vi "configure stimulation dialog (subVI).vi"(7 "default directory (none)":path, 8 "error in (no error)":errorcluster, 9 "use initial config? (F)":bool, 10 "odor and manifold config":T1, 11 "initial stim. config [] (empty array)":T11 {"right odor"."port-odor ring" items=["off"=0, "fish water, 3 <Odor:3, Port:0>"=3, "alarm substance <Odor:5, Port:1>"=5]; "middle odor"."port-odor ring" items=["off"=0, "fish water, 2 <Odor:2, Port:0>"=2]; "left odor"."port-odor ring" items=["off"=0, "fish water, 1 <Odor:1, Port:0>"=1, "alanine <Odor:4, Port:1>"=4]; "duration, s" format="%.1f"}) -> (0 "error out":errorcluster, 2 "operation failed?":bool, 3 "stim. config [] out":T11 {"right odor"."port-odor ring" items=["off"=0, "fish water, 3 <Odor:3, Port:0>"=3, "alarm substance <Odor:5, Port:1>"=5]; "middle odor"."port-odor ring" items=["off"=0, "fish water, 2 <Odor:2, Port:0>"=2]; "left odor"."port-odor ring" items=["off"=0, "fish water, 1 <Odor:1, Port:0>"=1, "alanine <Odor:4, Port:1>"=4]; "duration, s" format="%.1f"})   [LabVIEW 2021]
uses:
  type-defs/stimulation configuration array (type def).ctl
  type-defs/stimulator configuration line cluster (type def).ctl
  type-defs/port-odor with color cluster (type def).ctl
  type-defs/port-odor ring (type def).ctl
  type-defs/odor color (type def).ctl
  type-defs/odor and manifold config cluster (type def).ctl
  type-defs/manifold configuration cluster array (type def).ctl
  type-defs/manifold configuration cluster (type def).ctl
  type-defs/manifold selection.ctl
  type-defs/single port single odor cluster.ctl
  type-defs/port number (type def).ctl
  type-defs/odor selection (type def).ctl
  type-defs/odor description array (type def).ctl
  type-defs/odor info cluster (type def).ctl
  type-defs/stimulation config UI states (type def).ctl
  type-defs/project_custom_error_codes_ring (type def).ctl
  <vilib>/Utility/error.llb/DialogType.ctl
  global-variables/global variables.vi
  <vilib>/Utility/error.llb/Error Cluster From Error Code.vi
  <vilib>/ErrorRing/Error Ring.xnode
panel:
  in  "stim. config array dialog":T11 caption="Configure Odor Stimulation Sequence" {"right odor"."port-odor ring" items=["off"=0, "fish water, 3 (Odor: 3, Port: R.1)"=3, "alarm substance (Odor: 5, Port: R.2)"=5]; "middle odor"."port-odor ring" items=["off"=0, "fish water, 2 (Odor: 2, Port: M.1)"=2]; "left odor"."port-odor ring" items=["off"=0, "fish water, 1 (Odor: 1, Port: L.1)"=1, "alanine (Odor: 4, Port: L.2)"=4]; "duration, s" format="%.1f"}
  out "value error source":string
  in  "load config":bool
  in  "save config":bool
  in  "confirm button":bool
  in  "cancel button":bool
  # "description"
  # "duration, s"
  # "left"
  # "middle"
  # "right"
  # "File"
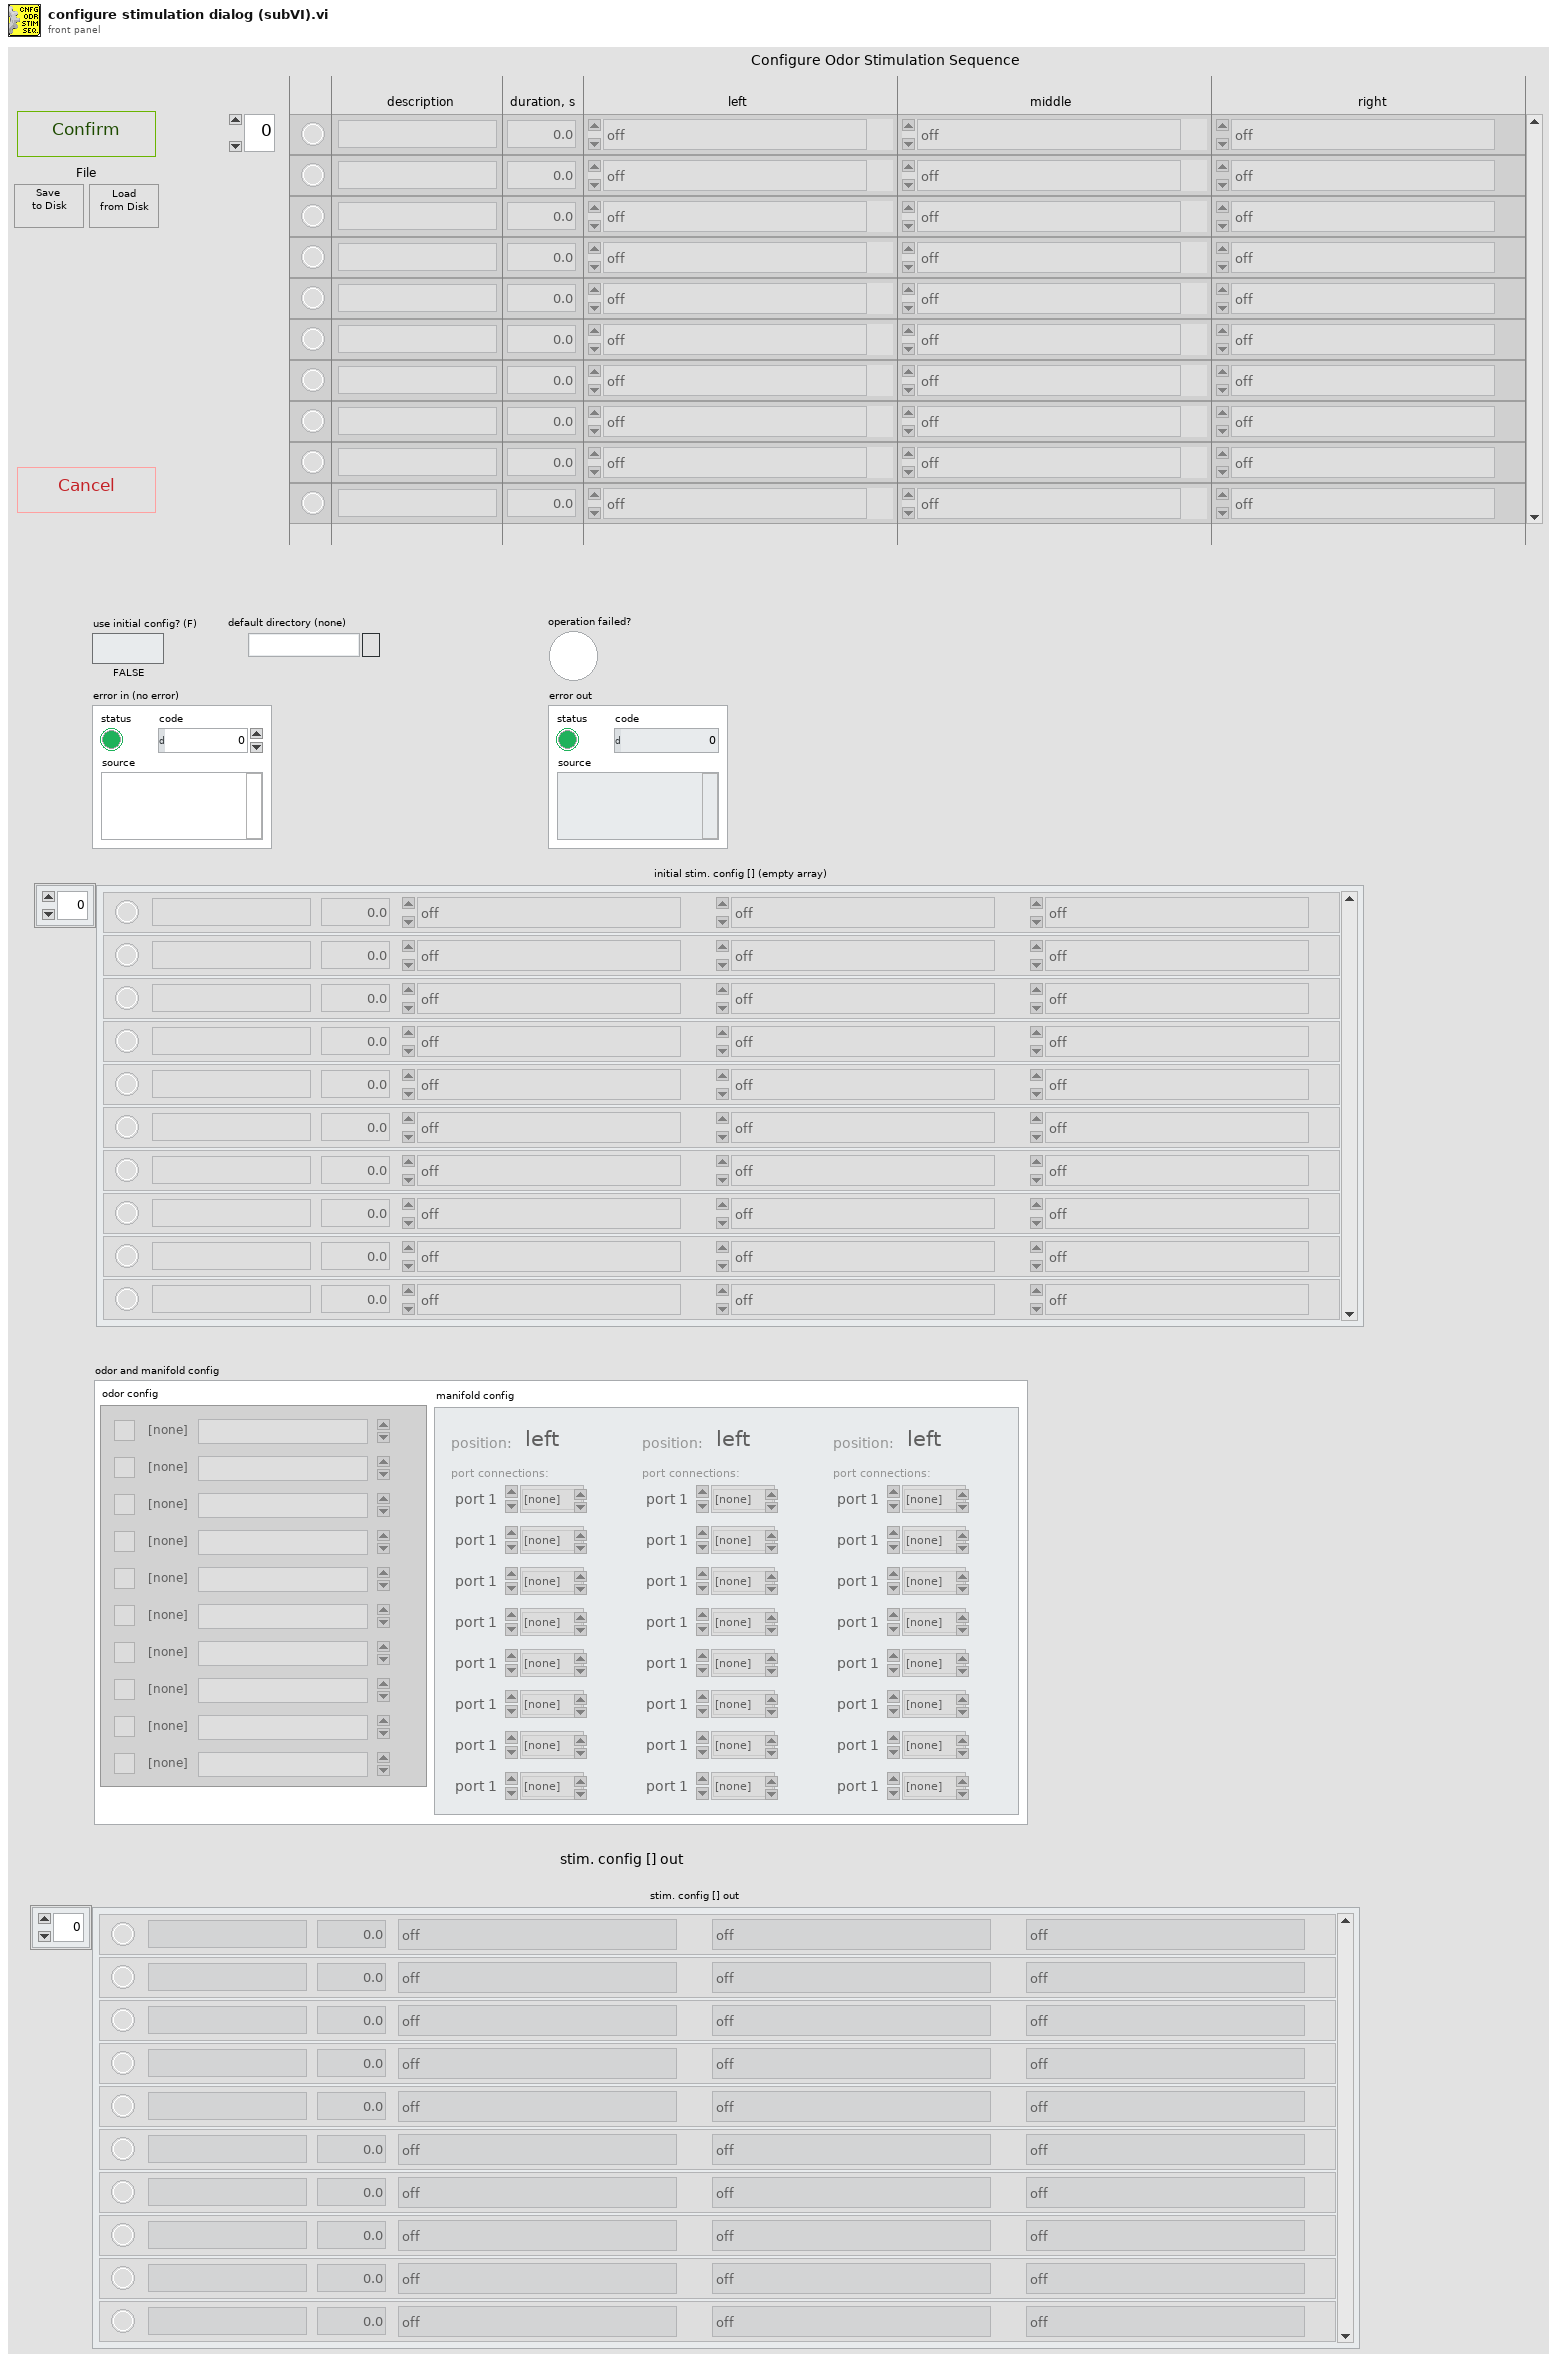
[diagram p1: front panel]
types:
  T1 = typedef "odor and manifold config cluster (type def).ctl" = cluster{"manifold config":T2, "odor config":T9}
  T2 = typedef "manifold configuration cluster array (type def).ctl" = T3[]
  T3 = typedef "manifold configuration cluster (type def).ctl" = cluster{"position:":T4, "port connections:":T5[]}
  T4 = typedef "manifold selection.ctl" = enum16{"left", "middle", "right"}
  T5 = typedef "single port single odor cluster.ctl" = cluster{"port number":T6, "connected odor":T7, "error":bool, "odor color":T8}
  T6 = typedef "port number (type def).ctl" = enum16{"port 1", "port 2", "port 3", "port 4", "port 5", "port 6", "port 7", "port 8"}
  T7 = typedef "odor selection (type def).ctl" = enum16{"[none]", "odor 1", "odor 2", "odor 3", "odor 4", "odor 5", "odor 6", "odor 7", "odor 8", "odor 9", "odor 10"}
  T8 = typedef "odor color (type def).ctl" = u16
  T9 = typedef "odor description array (type def).ctl" = T10[]
  T10 = typedef "odor info cluster (type def).ctl" = cluster{"odor channel":T7, "odor description":string, "odor color":T8, "odor channel active":bool}
  T11 = typedef "stimulation configuration array (type def).ctl" = T12[]
  T12 = typedef "stimulator configuration line cluster (type def).ctl" = cluster{"description":string, "duration, s":dbl, "left odor":T13, "middle odor":T13, "right odor":T13, "selected?":bool}
  T13 = typedef "port-odor with color cluster (type def).ctl" = cluster{"port-odor ring":T14, "odor color":T8}
  T14 = typedef "port-odor ring (type def).ctl" = u16
  T15 = typedef "stimulation config UI states (type def).ctl" = enum16{"Initialize", "Wait For Event", "Open Odor-Manifold Dialog", "Update Stim Config", "Handle Errors", "Save Config to File", "Load Config from File", "Exit", "Crash"}
  T16 = enum8{"Enabled", "Disabled", "Disabled and Grayed Out"}
  T17 = enum16{"open", "replace", "create", "open or create", "replace or create", "replace or create with confirmation"}
  T18 = enum16{"big-endian, network order", "native, host order", "little-endian"}
  T19 = cluster{"stim. config line cluster":refnum<vi>, "description string":refnum<vi>, "duration, s numeric":refnum<vi>, "port-odor & color cluster []":refnum<vi>[], "port-odor ring []":refnum<vi>[], "odor color ring []":refnum<vi>[]}
  T20 = typedef "project_custom_error_codes_ring (type def).ctl" = i32
  T21 = typedef "DialogType.ctl" = u16
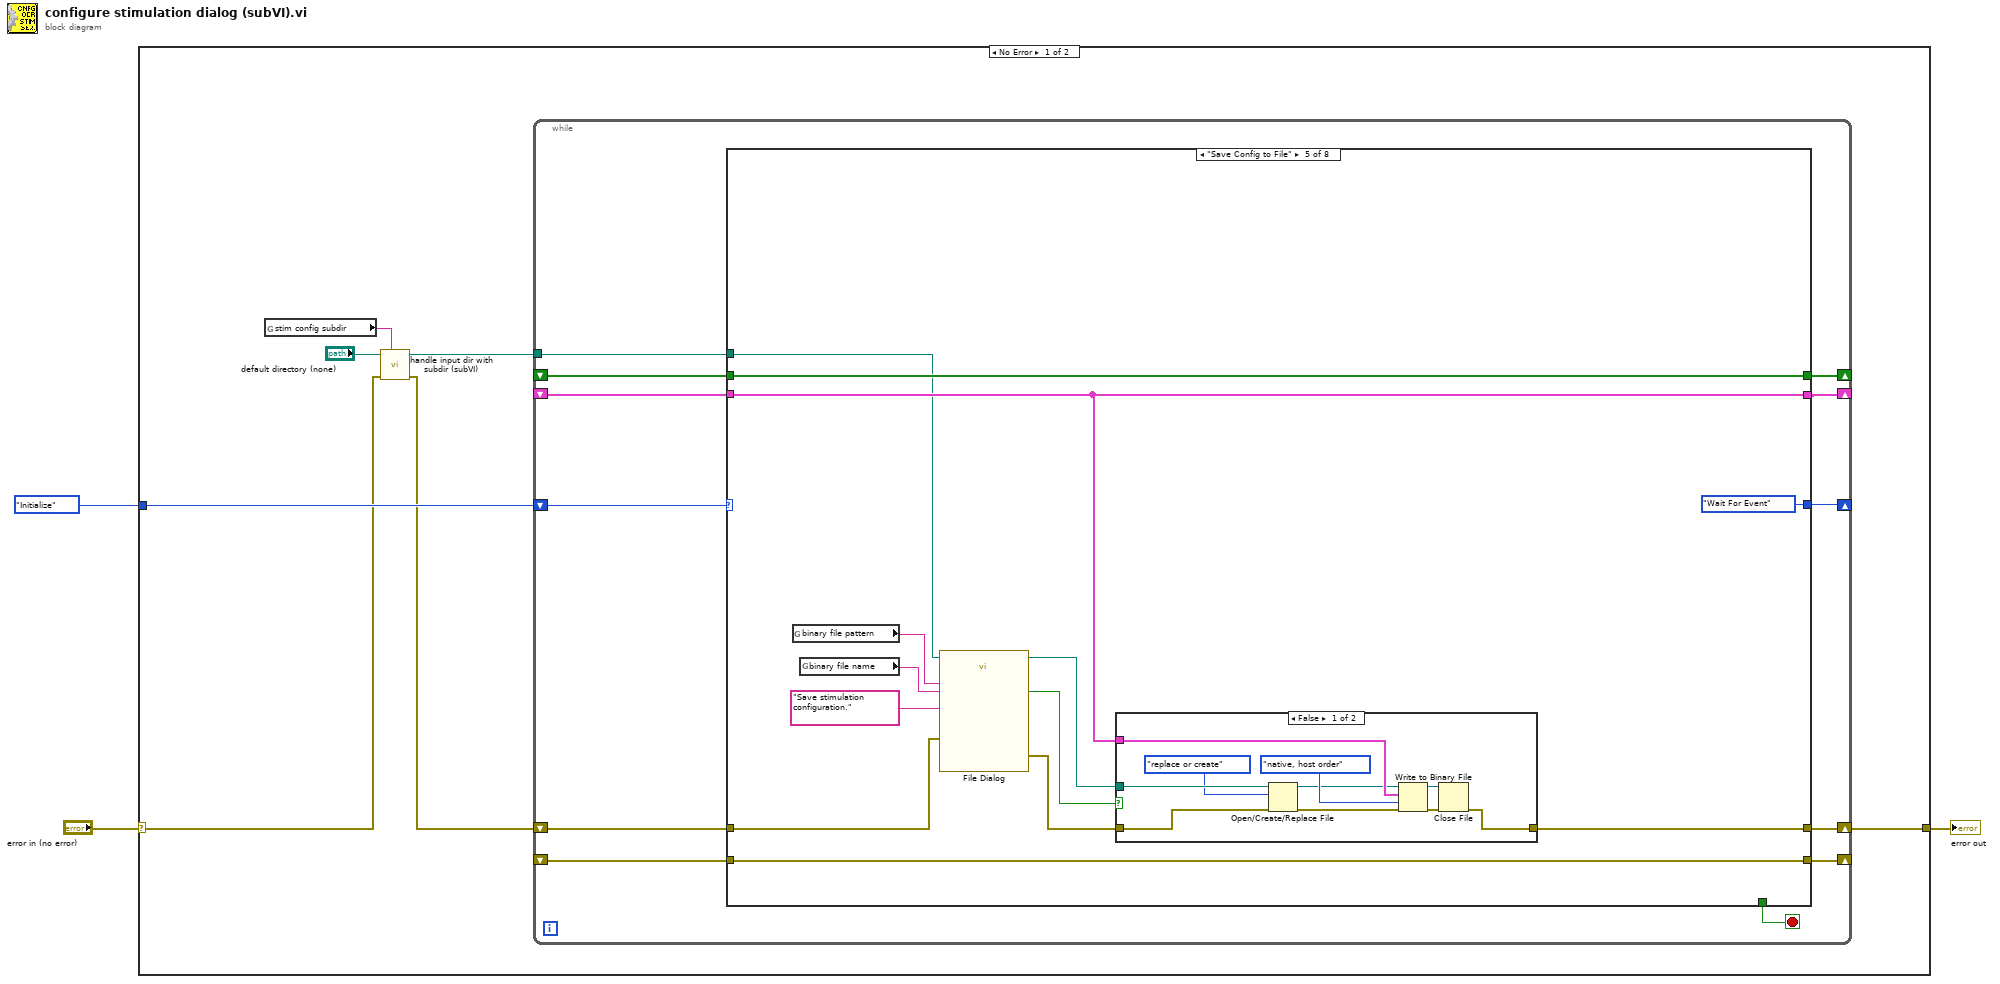
[diagram p0: block diagram]
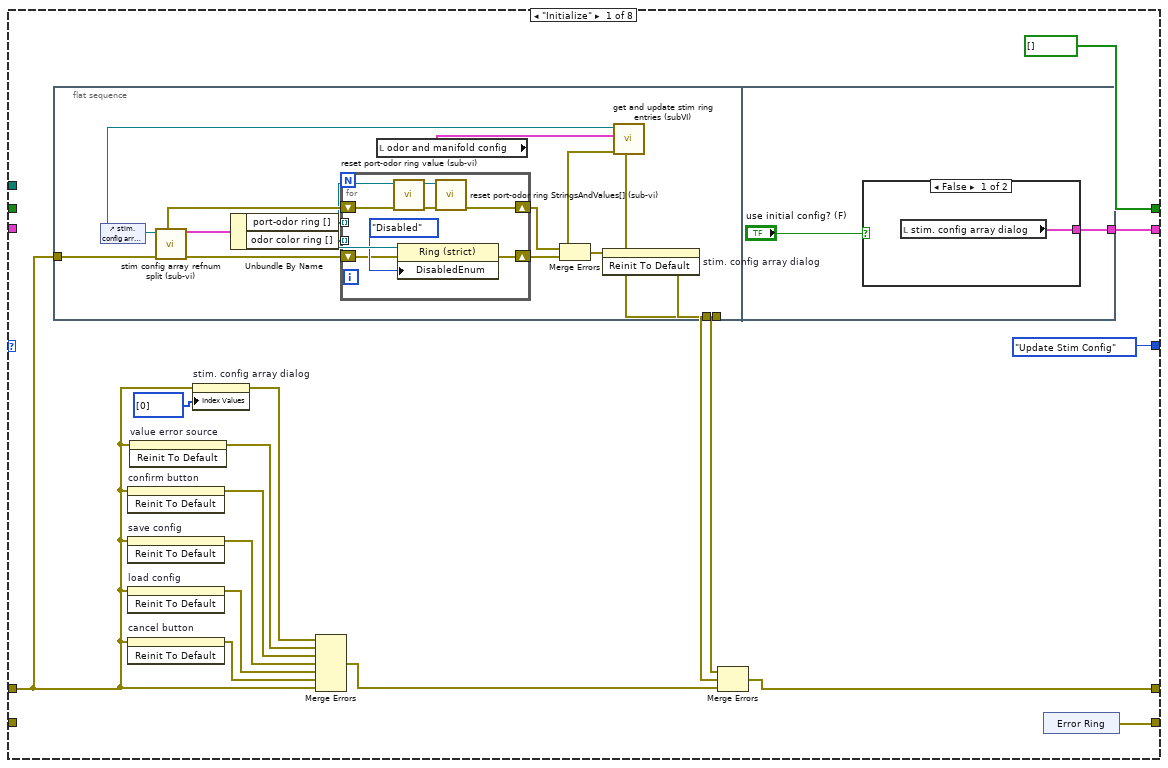
[diagram p2: hidden frame]
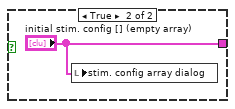
[diagram p3: hidden frame]
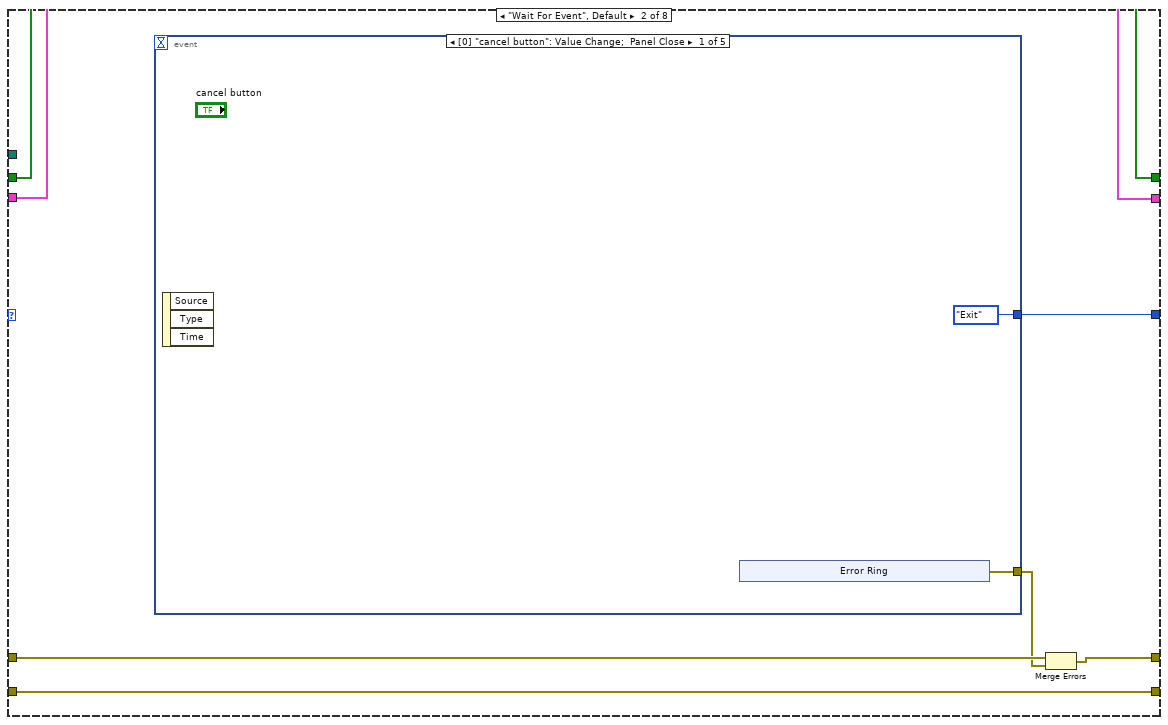
[diagram p4: hidden frame]
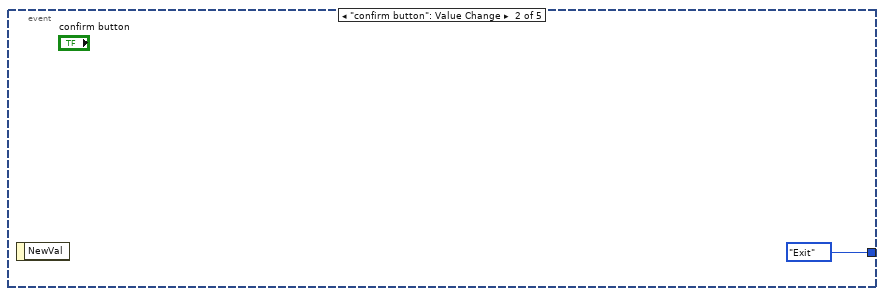
[diagram p5: hidden frame]
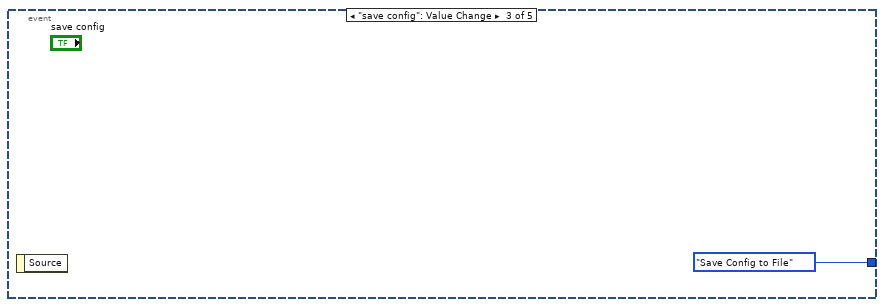
[diagram p6: hidden frame]
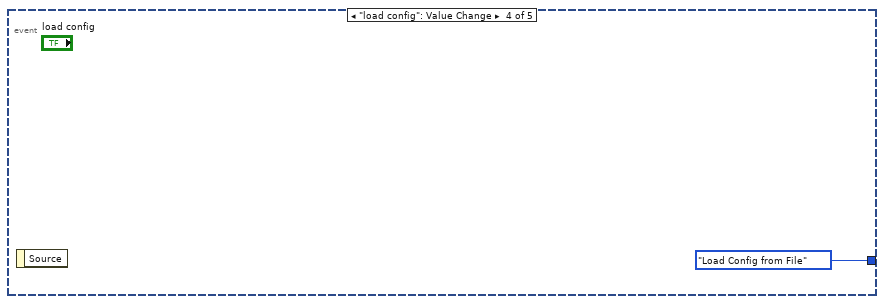
[diagram p7: hidden frame]
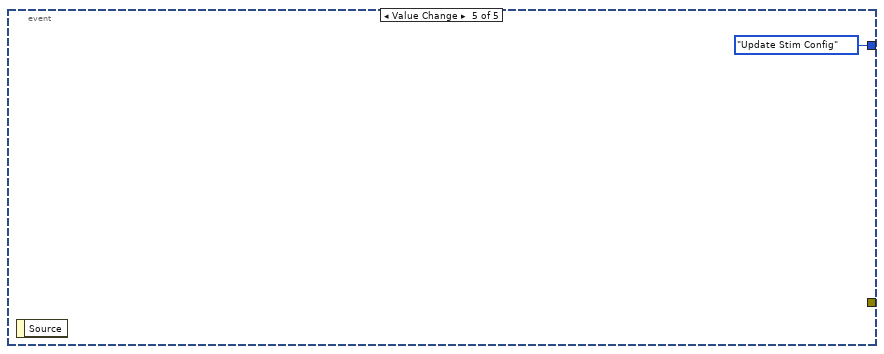
[diagram p8: hidden frame]
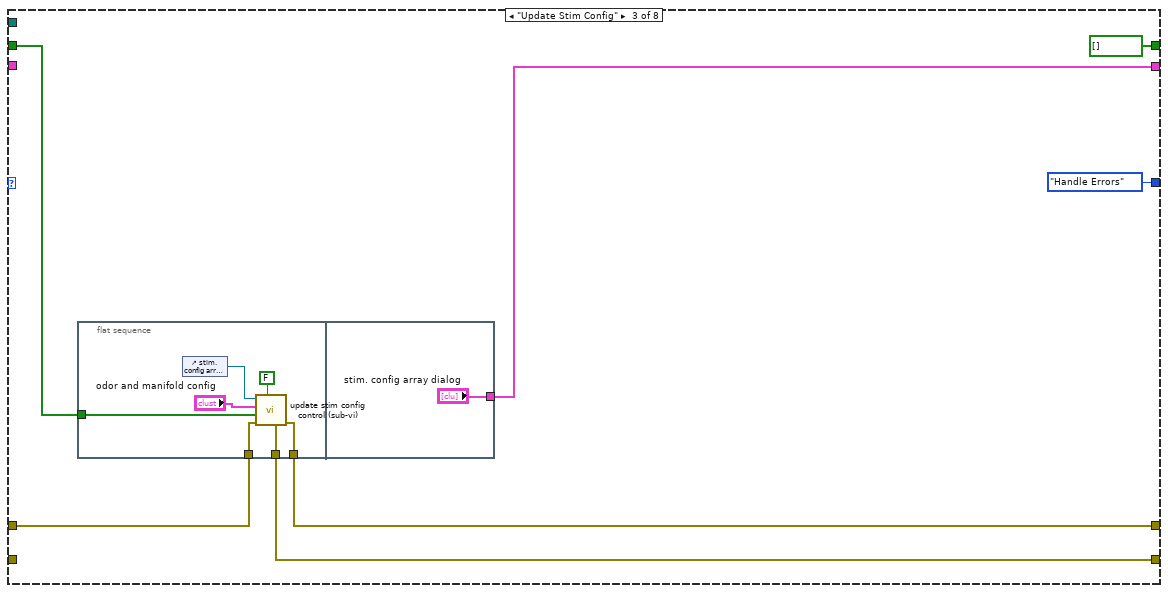
[diagram p9: hidden frame]
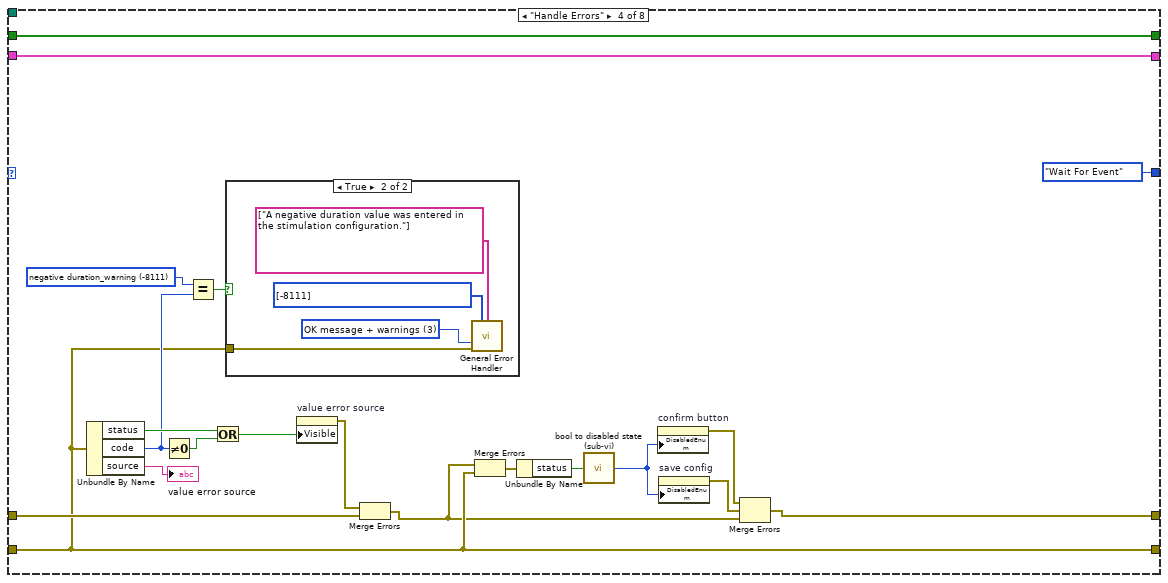
[diagram p10: hidden frame]
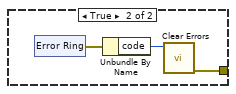
[diagram p12: hidden frame]
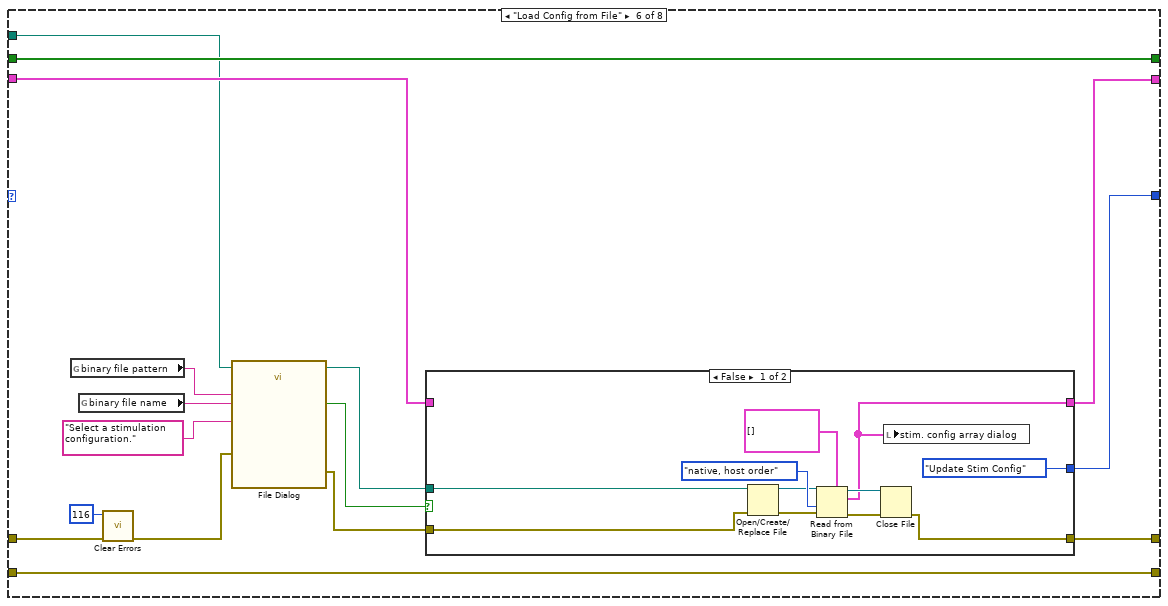
[diagram p13: hidden frame]
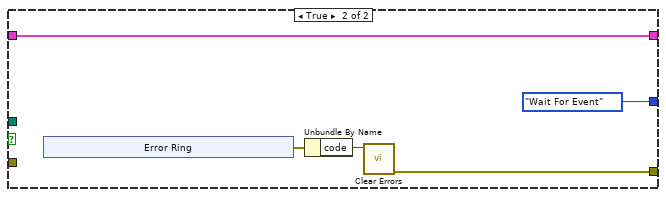
[diagram p14: hidden frame]
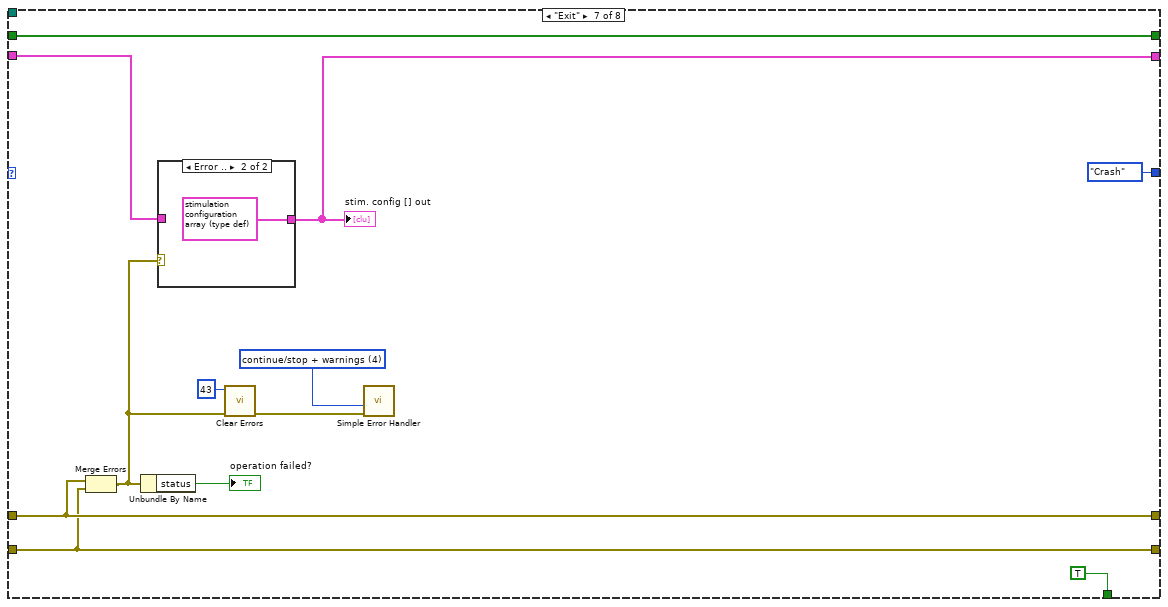
[diagram p15: hidden frame]
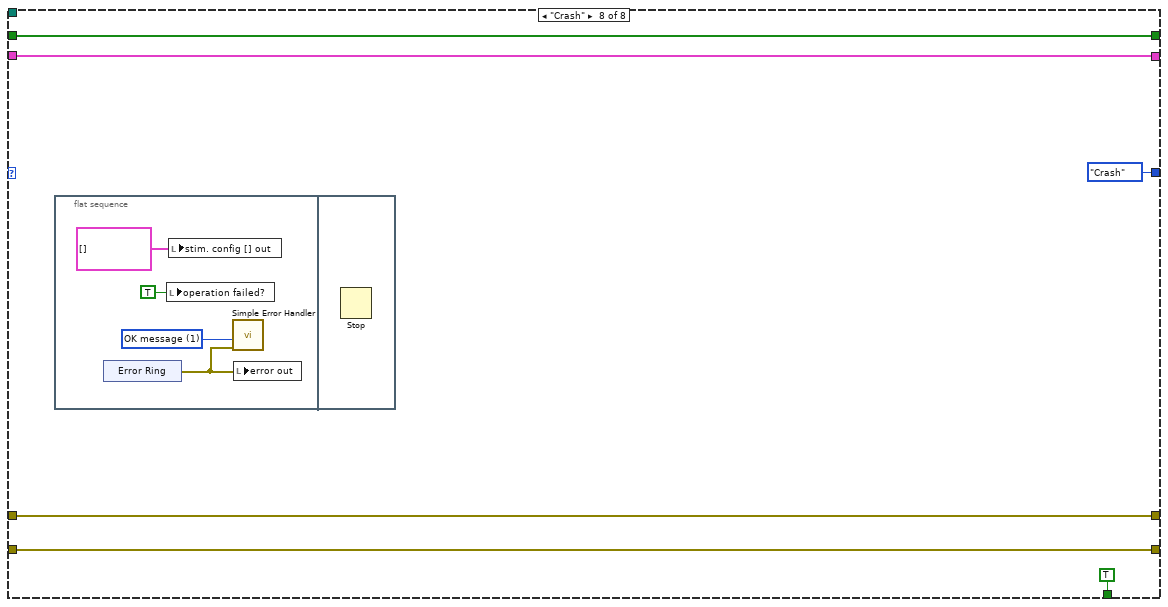
[diagram p17: hidden frame]
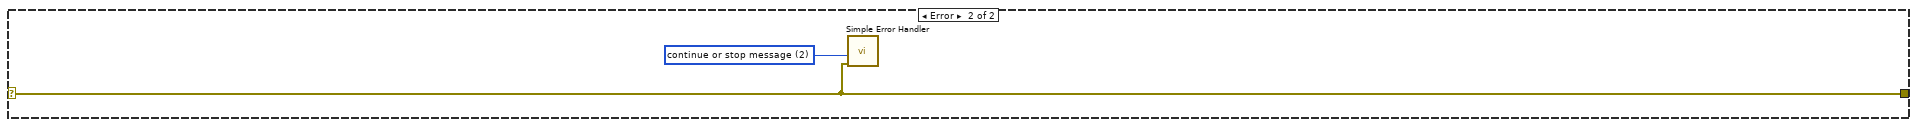
[diagram p18: hidden frame]
diagram:
  n1 = case shown="No Error" "error in (no error)" {
    selector: "error in (no error)" -> [w6 w216]
    tunnel: [w10 w216] -> w2
    tunnel: stimulation_config_UI_states_(type_def)."Initialize" ("Enum") -> [w9 _]
    frame No Error {
      n2 = global read "global variables.vi" "stim config subdir"() -> (w8:string)
      n3 = call "handle input dir with subdir (subVI).vi"("subdir name (none)"=w8, "error in (no error)"=w6, "starting directory (none)"="default directory (none)") -> ("error out"=w5:errorcluster, "dirctory path"=w4:path)  [unwired: 7 in]
      n4 = while {
        shift-right: [w20] -> _
        shift-left: w9 -> [w22]
        shift-right: [w21] -> w10
        shift-left: w5 -> [w18]
        shift-right: [w19] -> _
        shift-left: _ -> [w17]
        shift-right: [w16] -> _
        shift-left: _ -> [w15]
        shift-right: [w14] -> _
        shift-left: _ -> [w13]
        tunnel: w4 -> [w11]
        stop <- w12 stop-if-true
        n5 = case shown="\"Save Config to File\"" w22 {
          tunnel: w18 -> [w24 w66 w88 w113 w125 w160 w193 w202]
          tunnel: [w31 w69 w87 w102 w132 w166 w193 w202] -> w21
          tunnel: [stimulation_config_UI_states_(type_def)."Update Stim Config" ("Enum") w68 stimulation_config_UI_states_(type_def)."Handle Errors" ("Enum") stimulation_config_UI_states_(type_def)."Wait For Event" ("Enum") stimulation_config_UI_states_(type_def)."Wait For Event" ("Enum") w165 stimulation_config_UI_states_(type_def)."Crash" ("Enum") stimulation_config_UI_states_(type_def)."Crash" ("Enum")] -> w20
          tunnel: [w30 w67 w86 w104 w133 w161 w192 w201] -> w19
          tunnel: w17 -> [_ w67 _ w104 w133 w161 w192 w201]
          tunnel: [w29 w70 w85 w110 w131 w164 w191 w206] -> w16
          tunnel: w15 -> [_ w70 _ w110 w131 w162 w195 w206]
          tunnel: [bool[] [] w71 bool[] [] w109 w130 w163 w197 w205] -> w14
          tunnel: w13 -> [_ w71 w84 w109 w130 w163 w197 w205]
          tunnel: [_ _ _ _ _ _ TRUE TRUE] -> w12
          tunnel: w11 -> [_ _ _ _ w121 w157 _ _]
          frame "Initialize" {
            n6 = flat-sequence {
              tunnel: [w45] -> w33
              tunnel: w24 -> [w44]
              tunnel: [w40] -> w23
              tunnel: [w61] -> w29
              frame #0 {
                n7 = control-ref of="stim. config array dialog"() -> (w42:refnum<vi>)
                n8 = call "stim config array refnum split (sub-vi).vi"("error in (no error)"=w44, "stim. config array refnum"=w42) -> ("error out"=w48:errorcluster, "element refnum cluster"=w51:T19)  [unwired: 7 in, 1 out]
                n9 = Unbundle By Name(w51) -> ("port-odor ring []"=w49:refnum<vi>[], "odor color ring []"=w50:refnum<vi>[])
                n10 = for {
                  tunnel: w50 -> [w60] mode=indexing
                  shift-right: [w57] -> w47
                  shift-left: w48 -> [w58]
                  tunnel: w49 -> [w54] mode=indexing
                  shift-right: [w52] -> w46
                  shift-left: w48 -> [w53]
                  n11 = call "reset port-odor ring value (sub-vi).vi"("error in (no error)"=w53, "port-odor ring refnum"=w54) -> ("error out"=w56:errorcluster, "port-odor ring refnum out"=w55:refnum<vi>)  [unwired: 8 in]
                  n12 = property class="Ring (strict)"(reference=w60, error in=w58, "DisabledEnum"=T16."Disabled" ("Disabled")) -> (error out=w57:errorcluster)  [unwired: 1 out]
                  n13 = call "reset port-odor ring StringsAndValues[] (sub-vi).vi"("error in (no error)"=w56, "port-odor ring refnum"=w55) -> ("error out"=w52:errorcluster)  [unwired: 8 in, 1 out]
                }
                n14 = local read "odor and manifold config"() -> (w41:T1)
                n15 = Merge Errors(w46, w47) -> (w43:errorcluster)
                n16 = invoke on="stim. config array dialog" class="Arr (strict)" method="Reinit To Default"(error in=w43) -> (error out=w45:errorcluster)  [unwired: 2 in, 2 out]
                n17 = call "get and update stim ring entries (subVI).vi"("error in (no error)"=w43, "odor-manifold config"=w41, "stim config array refnum"=w42) -> ("error out"=w40:errorcluster)  [unwired: 7 in, 1 out]
              }
              frame #1 {
                n18 = case shown="False" "use initial config? (F)" {
                  tunnel: [w63 "initial stim. config [] (empty array)"] -> w61
                  frame False {
                    n19 = local read "stim. config array dialog"() -> (w63:T11)
                  }
                  frame True {
                    n20 = local write "stim. config array dialog"("initial stim. config [] (empty array)") -> ()
                  }
                }
              }
            }
            n21 = invoke on="confirm button" class="Bool" method="Reinit To Default"(error in=w24) -> (error out=w37:errorcluster)  [unwired: 2 in, 2 out]
            n22 = invoke on="save config" class="Bool" method="Reinit To Default"(error in=w24) -> (error out=w36:errorcluster)  [unwired: 2 in, 2 out]
            n23 = invoke on="load config" class="Bool" method="Reinit To Default"(error in=w24) -> (error out=w35:errorcluster)  [unwired: 2 in, 2 out]
            n24 = invoke on="cancel button" class="Bool" method="Reinit To Default"(error in=w24) -> (error out=w34:errorcluster)  [unwired: 2 in, 2 out]
            n25 = invoke on="value error source" class="Str" method="Reinit To Default"(error in=w24) -> (error out=w27:errorcluster)  [unwired: 2 in, 2 out]
            n26 = property on="stim. config array dialog" class="Arr (strict)"(error in=w24, "Index Values"=u32[] [0]) -> (error out=w25:errorcluster)  [unwired: 1 in, 1 out]
            n27 = Merge Errors(w25, w27, w37, w36, w35, w34, w24) -> (w32:errorcluster)
            n28 = Merge Errors(w23, w33, w32) -> (w31:errorcluster)
            n29 = xnode "Error Ring"() -> ("error out"=w30:errorcluster)
          }
          frame "Wait For Event", Default {
            n30 = event shown="[0] \"cancel button\": Value Change;  Panel Close" {
              selector: _ -> [_ _ _ _ _]
              dyn-events: _ -> [_ _ _ _ _]
              timeout: _ -> [_ _ _ _ _]
              tunnel: [w73 _ _ _ _] -> w65
              tunnel: [stimulation_config_UI_states_(type_def)."Exit" ("Enum") stimulation_config_UI_states_(type_def)."Exit" ("Enum") stimulation_config_UI_states_(type_def)."Save Config to File" ("Enum") stimulation_config_UI_states_(type_def)."Load Config from File" ("Enum") stimulation_config_UI_states_(type_def)."Update Stim Config" ("Enum")] -> w68
              event "cancel button": Value Change; Panel Close {
                n31 = event-data() -> ()  [unwired: 1 in, 3 out]
                n32 = xnode "Error Ring"() -> ("error out"=w73:errorcluster)
              }
              event "confirm button": Value Change {
                n33 = event-data() -> ()  [unwired: 1 in, 1 out]
              }
              event "save config": Value Change {
                n34 = event-data() -> ()  [unwired: 1 in, 1 out]
              }
              event "load config": Value Change {
                n35 = event-data() -> ()  [unwired: 1 in, 1 out]
              }
              event Value Change {
                n36 = event-data() -> ()  [unwired: 1 in, 1 out]
              }
            }
            n37 = Merge Errors(w66, w65) -> (w69:errorcluster)
          }
          frame "Update Stim Config" {
            n38 = flat-sequence {
              tunnel: w88 -> [w94]
              tunnel: [w93] -> w87
              tunnel: [w92] -> w86
              tunnel: w84 -> [w91]
              tunnel: ["stim. config array dialog"] -> w85
              frame #0 {
                n39 = control-ref of="stim. config array dialog"() -> (w95:refnum<vi>)
                n40 = call "update stim config control (sub-vi).vi"("update ring entries? (T)"=FALSE, "error in (no error)"=w94, "changed? [] (empty)"=w91, "odor-manifold config"="odor and manifold config", "stim. config array refnum"=w95) -> ("error out"=w93:errorcluster, "value error"=w92:errorcluster)  [unwired: 4 in, 1 out]
              }
              frame #1 {
              }
            }
          }
          frame "Handle Errors" {
            w107 = T20 -8111 items=["parse_failure"=-8001, "arduino_failure"=-8002, "manifold_config_value_error"=-8101, "odor_config_value_error"=-8102, "negative duration_warning"=-8111] ("Ring")
            n41 = Unbundle By Name(w104) -> ("status"=w115:bool, "code"=w106:i32, "source"=→"value error source":string)
            n42 = Not Equal To 0?(x=w106) -> (x != 0?=w116:bool)
            n43 = Equal?(x=w107, y=w106) -> (x = y?=w105:bool)
            n44 = Or(x=w115, y=w116) -> (x .or. y?=w112:bool)
            n45 = case shown="True" w105 {
              tunnel: w104 -> [_ w117]
              frame False {
              }
              frame True {
                w119 = T20[] [-8111] items=["parse_failure"=-8001, "arduino_failure"=-8002, "manifold_config_value_error"=-8101, "odor_config_value_error"=-8102, "negative duration_warning"=-8111] ("[user-defined codes]")
                w120 = T21 3 items=["no dialog", "OK message", "continue or stop message", "OK message + warnings", "continue/stop + warnings"] ("type of dialog (OK msg:1)")
                n46 = call <vilib>:"General Error Handler.vi"("[user-defined codes]"=w119, "[user-defined descriptions]"=string[] ["A negative duration value was entered in the stimulation configuration."], "type of dialog (OK msg:1)"=w120, "error in (no error)"=w117) -> ()  [unwired: 7 in, 5 out]
              }
            }
            n47 = property on="value error source" class="Str"("Visible"=w112) -> (error out=w111:errorcluster)  [unwired: 2 in, 1 out]
            n48 = Merge Errors(w111, w113) -> (w103:errorcluster)
            n49 = Merge Errors(w103, w104) -> (w99:errorcluster)
            n50 = Unbundle By Name(w99) -> ("status"=w98:bool)
            n51 = call "bool to disabled state (sub-vi).vi"("error?"=w98) -> ("disabled"=w97:T16)
            n52 = property on="confirm button" class="Bool"("DisabledEnum"=w97) -> (error out=w100:errorcluster)  [unwired: 2 in, 1 out]
            n53 = property on="save config" class="Bool"("DisabledEnum"=w97) -> (error out=w101:errorcluster)  [unwired: 2 in, 1 out]
            n54 = Merge Errors(w100, w101, w103) -> (w102:errorcluster)
          }
          frame "Save Config to File" {
            n55 = global read "global variables.vi" "binary file pattern"() -> (w127:string)
            n56 = global read "global variables.vi" "binary file name"() -> (w128:string)
            n57 = call "File Dialog"("start path"=w121, "prompt"="Save stimulation configuration.", "error in"=w125, "pattern (all files)"=w127, "pattern label"=w128) -> ("selected path"=w122:path, "cancelled"=w123:bool, "error out"=w124:errorcluster)  [unwired: 7 in, 1 out]
            n58 = case shown="False" w123 {
              tunnel: [w140 w144] -> w132
              tunnel: w131 -> [w139 _]
              tunnel: w124 -> [w138 _]
              tunnel: w122 -> [w135 _]
              frame False {
                n59 = Open/Create/Replace File(file path (use dialog)=w135, error in=w138, operation (0:open)=T17."replace or create") -> (refnum out=w136:refnum<file>, error out=w137:errorcluster)  [unwired: 3 in, 1 out]
                n60 = Write to Binary File(file (use dialog)=w136, data=w139, error in=w137, 9:T18."native, host order" ("byte order (0:big-endian, network order)")) -> (refnum out=w142:refnum<file>, error out=w143:errorcluster)  [unwired: 2 in, 1 out]
                n61 = Close File(refnum=w142, error in=w143) -> (error out=w140:errorcluster)  [unwired: 1 out]
              }
              frame True {
                n62 = xnode "Error Ring"() -> ("error out"=w146:errorcluster)
                n63 = Unbundle By Name(w146) -> ("code"=w145:i32)
                n64 = call <vilib>:"Clear Errors.vi"("specific error code to clear (0: all)"=w145) -> ("error out"=w144:errorcluster)  [unwired: 5 in, 1 out]
              }
            }
          }
          frame "Load Config from File" {
            n65 = global read "global variables.vi" "binary file pattern"() -> (w154:string)
            n66 = global read "global variables.vi" "binary file name"() -> (w155:string)
            n67 = call <vilib>:"Clear Errors.vi"("error in (no error)"=w160, "specific error code to clear (0: all)"=116) -> ("error out"=w152:errorcluster)  [unwired: 4 in, 1 out]
            n68 = call "File Dialog"("start path"=w157, "prompt"="Select a stimulation configuration.", "error in"=w152, "pattern (all files)"=w154, "pattern label"=w155) -> ("selected path"=w153:path, "cancelled"=w158:bool, "error out"=w159:errorcluster)  [unwired: 7 in, 1 out]
            n69 = case shown="False" w158 {
              tunnel: [w174 w182] -> w166
              tunnel: [w172 w178] -> w164
              tunnel: [stimulation_config_UI_states_(type_def)."Update Stim Config" ("Enum") stimulation_config_UI_states_(type_def)."Wait For Event" ("Enum")] -> w165
              tunnel: w162 -> [_ w178]
              tunnel: w159 -> [w170 _]
              tunnel: w153 -> [w167 _]
              frame False {
                n70 = Open/Create/Replace File(file path (use dialog)=w167, error in=w170) -> (refnum out=w168:refnum<file>, error out=w169:errorcluster)  [unwired: 4 in, 1 out]
                n71 = Read from Binary File(5:T11 [] ("stim. config array dialog"), 8:w169, 9:T18."native, host order" ("byte order (0:big-endian, network order)"), 11:w168) -> (0:w177:errorcluster, 2:w172:T11, 3:w176:refnum<file>)  [unwired: 2 in, 1 out]
                n72 = Close File(refnum=w176, error in=w177) -> (error out=w174:errorcluster)  [unwired: 1 out]
                n73 = local write "stim. config array dialog"(w172) -> ()
              }
              frame True {
                n74 = xnode "Error Ring"() -> ("error out"=w181:errorcluster)
                n75 = Unbundle By Name(w181) -> ("code"=w180:i32)
                n76 = call <vilib>:"Clear Errors.vi"("specific error code to clear (0: all)"=w180) -> ("error out"=w182:errorcluster)  [unwired: 5 in, 1 out]
              }
            }
          }
          frame "Exit" {
            w187 = T21 4 items=["no dialog", "OK message", "continue or stop message", "OK message + warnings", "continue/stop + warnings"] ("type of dialog (OK msg:1)")
            n77 = Merge Errors(w193, w192) -> (w188:errorcluster)
            n78 = Unbundle By Name(w188) -> ("status"=→"operation failed?":bool)
            n79 = case shown="Error .." w188 {
              tunnel: w195 -> [w199 _]
              tunnel: [w199 T11 [{"description"="", "duration, s"=0.0, "left odor"={"port-odor ring"=0, "odor color"=9}, "middle odor"={"port-odor ring"=0, "odor color"=9}, "right odor"={"port-odor ring"=0, "odor color"=9}, "selected?"=FALSE}, {"description"="", "duration, s"=0.0, "left odor"={"port-odor ring"=0, "odor color"=9}, "middle odor"={"port-odor ring"=0, "odor color"=9}, "right odor"={"port-odor ring"=0, "odor color"=9}, "selected?"=FALSE}, {"description"="", "duration, s"=0.0, "left odor"={"port-odor ring"=0, "odor color"=9}, "middle odor"={"port-odor ring"=0, "odor color"=9}, "right odor"={"port-odor ring"=0, "odor color"=9}, "selected?"=FALSE}, {"description"="", "duration, s"=0.0, "left odor"={"port-odor ring"=0, "odor color"=9}, "middle odor"={"port-odor ring"=0, "odor color"=9}, "right odor"={"port-odor ring"=0, "odor color"=9}, "selected?"=FALSE}] ("stim. config array dialog")] -> w191
              frame No Error {
              }
              frame Error {
              }
            }
            "stim. config [] out" <- w191
            n80 = call <vilib>:"Clear Errors.vi"("error in (no error)"=w188, "specific error code to clear (0: all)"=43) -> ("error out"=w190:errorcluster)  [unwired: 4 in, 1 out]
            n81 = call <vilib>:"Simple Error Handler.vi"("type of dialog (OK msg:1)"=w187, "error in (no error)"=w190) -> ()  [unwired: 3 in, 5 out]
          }
          frame "Crash" {
            n82 = flat-sequence {
              frame #0 {
                w207 = T21 1 items=["no dialog", "OK message", "continue or stop message", "OK message + warnings", "continue/stop + warnings"] ("type of dialog (OK msg:1)")
                n83 = xnode "Error Ring"() -> ("error out"=w208:errorcluster)
                n84 = local write "operation failed?"(TRUE ("operation failed? 2")) -> ()
                n85 = local write "stim. config [] out"(T11 [] ("stim. config [] out")) -> ()
                n86 = call <vilib>:"Simple Error Handler.vi"("type of dialog (OK msg:1)"=w207, "error in (no error)"=w208) -> ()  [unwired: 3 in, 5 out]
                n87 = local write "error out"(w208) -> ()
              }
              frame #1 {
                n88 = Stop() -> ()  [unwired: 1 in]
              }
            }
          }
        }
      }
    }
    frame Error {
      w215 = T21 2 items=["no dialog", "OK message", "continue or stop message", "OK message + warnings", "continue/stop + warnings"] ("type of dialog (OK msg:1)")
      n89 = call <vilib>:"Simple Error Handler.vi"("type of dialog (OK msg:1)"=w215, "error in (no error)"=w216) -> ()  [unwired: 3 in, 5 out]
    }
  }
  "error out" <- w2
